vi "Script Editor.vi"(3 "error in (no error)":errorcluster) -> (0 "error out":errorcluster)   [LabVIEW 2011]
uses:
  Strict Type Controls/Settings Operation.ctl
  <userlib>/_OpenG.lib/comparison/comparison.llb/Boolean Changed__ogtk.vi
  Instance           1 21Saved   Script Editor .vi
  Instance           2 21Saved   Script Editor .vi
panel:
  out "Quit":bool
  in  "Update":bool
  in  "Remove":bool
  in  "Add":bool
  in  "Save As":bool
  in  "Save":bool
  in  "Open":bool
  in  "New":bool
  in  "Param 2":dbl
  in  "Param 1":dbl
  in  "Command":string(combo)
  in  "Comment":string
  in  "Script":i32(listbox)
  out "File Name":string
  out "Progress":u8(slide) scale=0.0..100.0
  # "App Designed For:"
  # "Web: www.jambhekar.com\nEmail: tushar@jambhekar.com\nCell: +919970168164"
  # "App Designed By:"
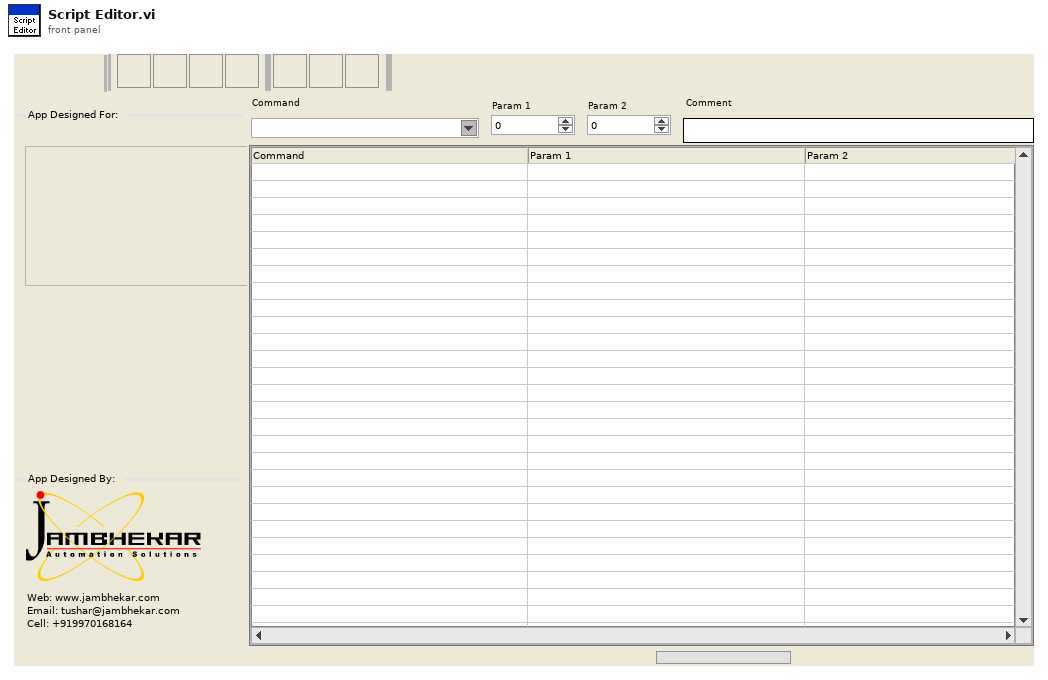
[diagram p1: front panel]
types:
  T1 = enum32{"Invalid", "Standard", "Closed", "Hidden", "Minimized", "Maximized"}
  T2 = typedef "Settings Operation.ctl" = enum8{"Get Value", "Set Value", "Read File", "Write File", "Write Stored Value"}
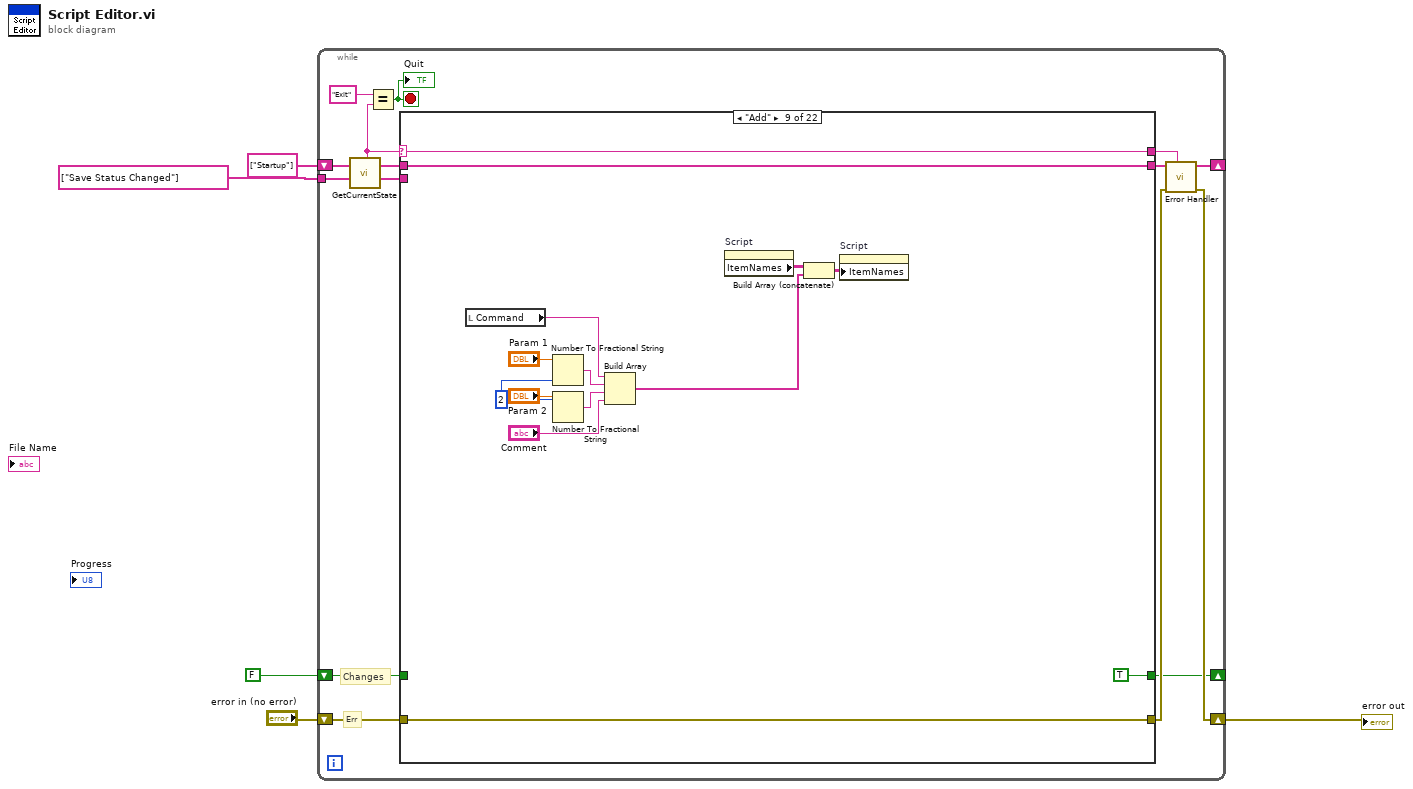
[diagram p0: block diagram]
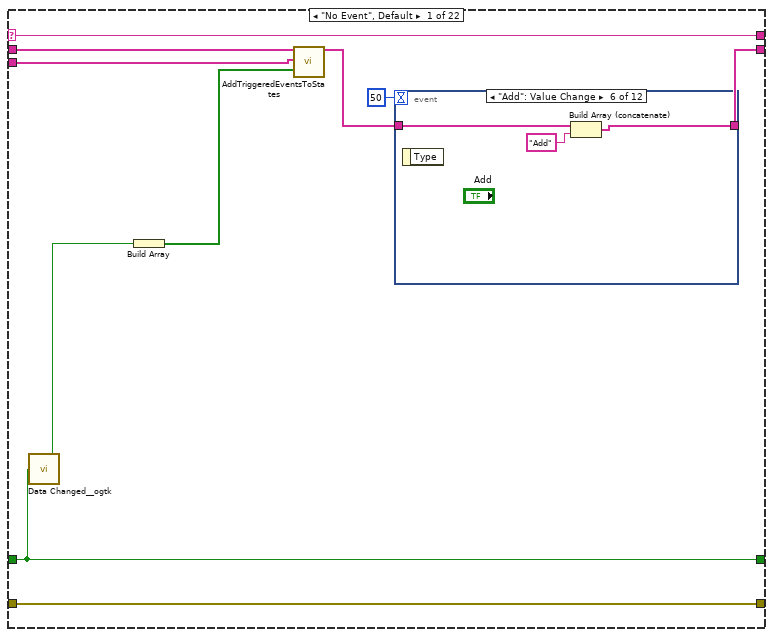
[diagram p2: hidden frame]
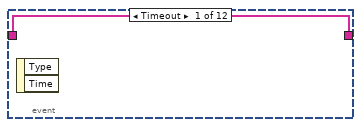
[diagram p3: hidden frame]
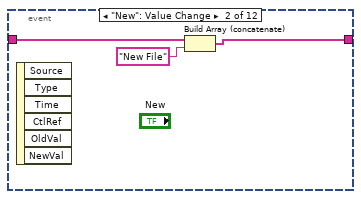
[diagram p4: hidden frame]
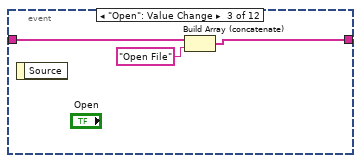
[diagram p5: hidden frame]
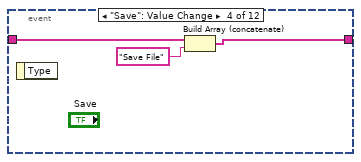
[diagram p6: hidden frame]
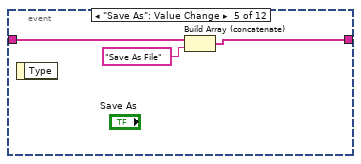
[diagram p7: hidden frame]
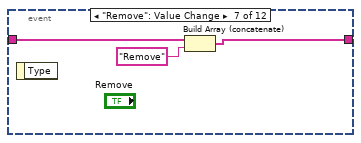
[diagram p8: hidden frame]
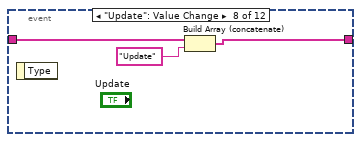
[diagram p9: hidden frame]
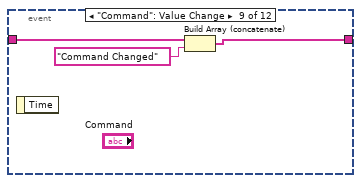
[diagram p10: hidden frame]
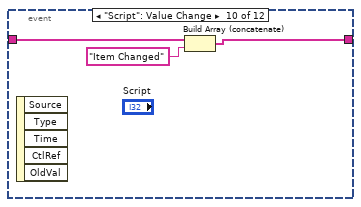
[diagram p11: hidden frame]
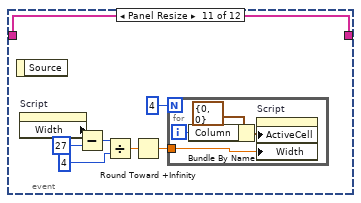
[diagram p12: hidden frame]
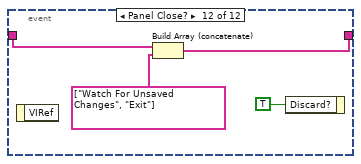
[diagram p13: hidden frame]
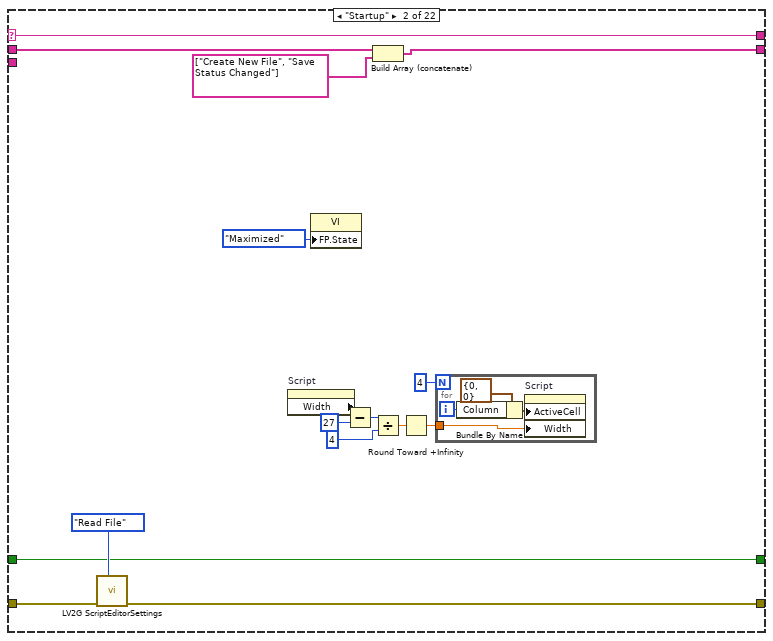
[diagram p14: hidden frame]
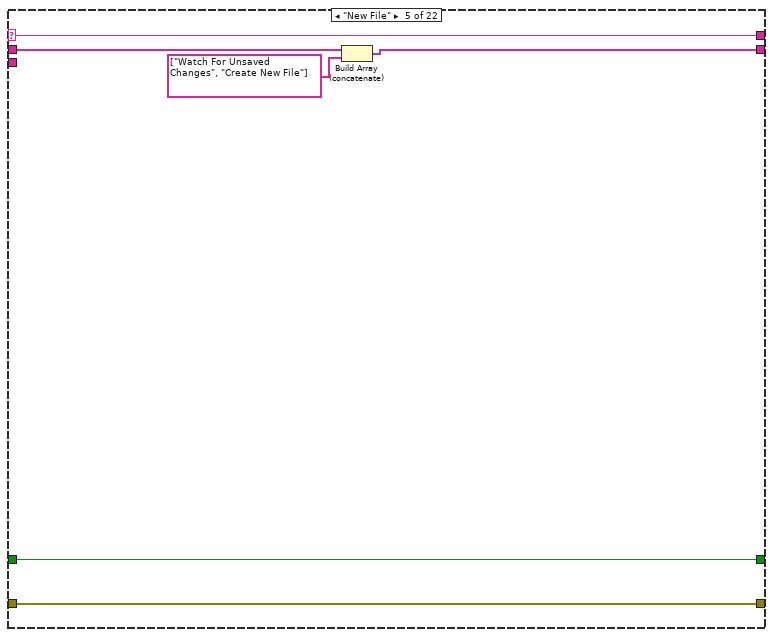
[diagram p17: hidden frame]
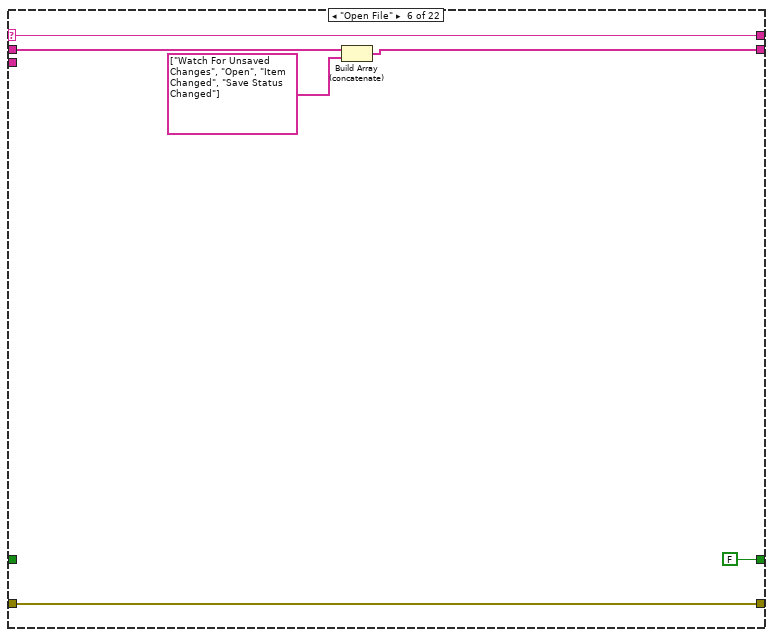
[diagram p18: hidden frame]
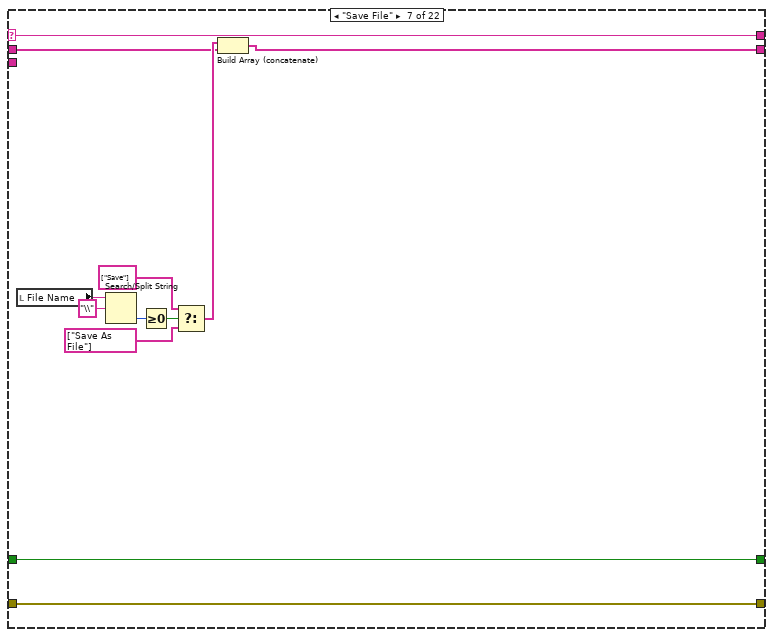
[diagram p19: hidden frame]
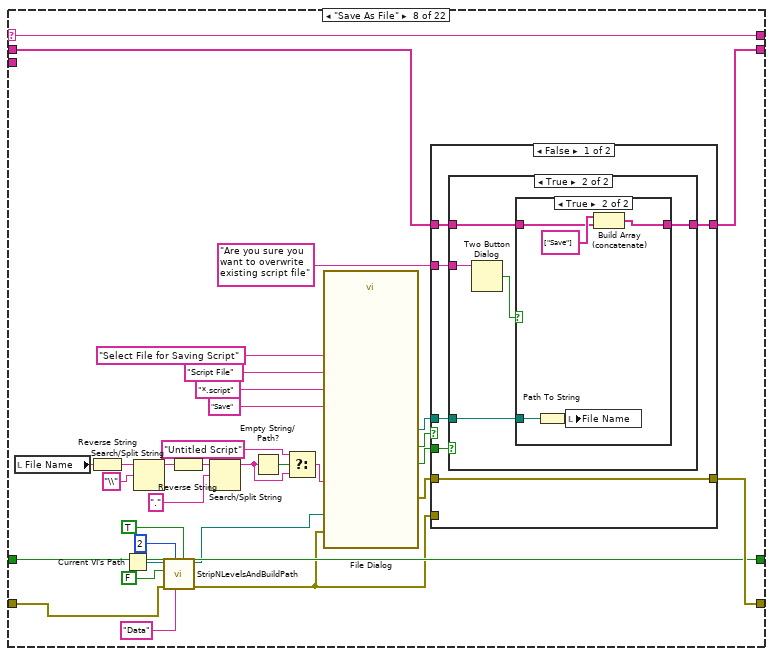
[diagram p20: hidden frame]
diagram:
  n1 = while {
    shift-right: [w13] -> _
    shift-left: string[] ["Startup"] ("State Array Out") -> [w19]
    tunnel: string[] ["Save Status Changed"] ("State Array Out") -> [w17]
    shift-right: [w10] -> w1
    shift-left: "error in (no error)" -> [w14]
    shift-right: [w7] -> _
    shift-left: FALSE -> [w8]
    stop <- w15 stop-if-true
    # "Changes"
    # "Err"
    n2 = call "GetCurrentState.vi"("State Array In"=w19) -> ("Current State"=w6:string, "State Array Out"=w18:string[])  [unwired: 1 in, 16 out]
    n3 = Equal?(x="Exit", y=w6) -> (x = y?=w15:bool)
    "Quit" <- w15
    n4 = case shown="\"Add\"" w6 {
      selector: w6 -> [w27 w89 w95 w99 w106 w112 w124 w157 w193 w206 w221 w226 w237 w243 w247 w253 w274 w279 w298 w317 w332 w336]
      tunnel: w18 -> [w29 w86 w97 w101 w103 w110 w116 w138 w195 w208 w223 w228 w234 w245 w249 w255 w266 w277 w291 w316 w331 w335]
      tunnel: [w22 w85 w97 w101 w102 w109 w115 w137 w195 w208 w223 w228 w233 w245 w249 w255 w265 w276 w290 w316 w331 w335] -> w12
      tunnel: w17 -> [w28 _ _ _ _ _ _ _ _ _ _ _ _ _ _ _ _ _ _ _ _ _]
      tunnel: [w26 w74 w96 w100 w107 w113 w125 w141 w194 w207 w222 w227 w238 w244 w248 w254 w271 w278 w297 w308 w330 errorcluster {"status"=FALSE, "code"=0, "source"=""} ("error in (no error)")] -> w9
      tunnel: w14 -> [w26 w75 w96 w100 w107 w113 w125 w128 w194 w207 w222 w227 w238 w244 w248 w254 w268 w278 w297 w301 w330 _]
      tunnel: [w27 w89 w95 w99 w106 w112 w124 w157 w193 w206 w221 w226 w237 w243 w247 w253 w274 w279 w298 w317 w332 w336] -> w11
      tunnel: w8 -> [w20 w87 w94 w98 w105 _ w114 w134 _ _ _ w225 w236 w242 w246 w251 _ w275 _ _ w329 w334]
      tunnel: [w20 w87 w94 w98 w105 FALSE w114 w134 TRUE TRUE TRUE w225 w236 w242 w246 w251 FALSE w275 FALSE FALSE w329 w334] -> w7
      frame "No Event", Default {
        n5 = call-poly <userlib>:"Data Changed__ogtk.vi"("Boolean"=w20) -> ("Changed"=w21:bool)
        n6 = Build Array(w21) -> (w25:bool[])
        n7 = call "AddTriggeredEventsToStates.vi"("State Array In"=w29, "Event List"=w28, "Event Triggers Array"=w25) -> ("State Array Out"=w23:string[])  [unwired: 16 out]
        n8 = event shown="[5] \"Add\": Value Change" {
          selector: _ -> [_ _ _ _ _ _ _ _ _ _ _ _]
          dyn-events: _ -> [_ _ _ _ _ _ _ _ _ _ _ _]
          timeout: 50 -> [_ _ _ _ _ _ _ _ _ _ _ _]
          tunnel: w23 -> [w30 w32 w35 w38 w41 w44 w47 w50 w53 w56 w59 w72]
          tunnel: [w30 w31 w34 w37 w40 w43 w46 w49 w52 w55 w59 w70] -> w22
          event Timeout {
            n9 = event-data() -> ()  [unwired: 3 out]
          }
          event "New": Value Change {
            n10 = event-data() -> ()  [unwired: 7 out]
            n11 = Build Array (concatenate)(w32, "New File" ("String")) -> (w31:string[])
          }
          event "Open": Value Change {
            n12 = event-data() -> ()  [unwired: 2 out]
            n13 = Build Array (concatenate)(w35, "Open File" ("String")) -> (w34:string[])
          }
          event "Save": Value Change {
            n14 = event-data() -> ()  [unwired: 2 out]
            n15 = Build Array (concatenate)(w38, "Save File" ("String")) -> (w37:string[])
          }
          event "Save As": Value Change {
            n16 = event-data() -> ()  [unwired: 2 out]
            n17 = Build Array (concatenate)(w41, "Save As File" ("String")) -> (w40:string[])
          }
          event "Add": Value Change {
            n18 = event-data() -> ()  [unwired: 2 out]
            n19 = Build Array (concatenate)(w44, "Add" ("String")) -> (w43:string[])
          }
          event "Remove": Value Change {
            n20 = event-data() -> ()  [unwired: 2 out]
            n21 = Build Array (concatenate)(w47, "Remove" ("String")) -> (w46:string[])
          }
          event "Update": Value Change {
            n22 = event-data() -> ()  [unwired: 2 out]
            n23 = Build Array (concatenate)(w50, "Update" ("String")) -> (w49:string[])
          }
          event "Command": Value Change {
            n24 = event-data() -> ()  [unwired: 2 out]
            n25 = Build Array (concatenate)(w53, "Command Changed" ("String")) -> (w52:string[])
          }
          event "Script": Value Change {
            n26 = event-data() -> ()  [unwired: 6 out]
            n27 = Build Array (concatenate)(w56, "Item Changed" ("String")) -> (w55:string[])
          }
          event Panel Resize {
            n28 = event-data() -> ()  [unwired: 2 out]
            n29 = property on="Script" class="MCListbox (strict)"() -> ("Width"=w60:u32)  [unwired: 2 in, 2 out]
            n30 = Subtract(x=w60, y=u32 27) -> (x-y=w62:u32)
            n31 = Divide(x=w62, y=u32 4) -> (x/y=w64:dbl)
            n32 = Round Toward +Infinity(x=w64) -> (ceil(x): smallest int >= x=w65:dbl)
            n33 = for {
              N: 4 -> [_]
              tunnel: w65 -> [w66]
              i -> [w68]
              n34 = Bundle By Name(cluster=cluster{"Row":i32, "Column":i32} {"Row"=0, "Column"=0} ("Active Cell:Active Cell"), "Column"=w68) -> (w67:cluster{"Row":i32, "Column":i32})
              n35 = property on="Script" class="MCListbox (strict)"("ActiveCell"=w67, "Width"=w66) -> ()  [unwired: 2 in, 2 out]
            }
          }
          event Panel Close? {
            n36 = event-data() -> ()  [unwired: 2 out]
            n37 = Build Array (concatenate)(w72, string[] ["Watch For Unsaved Changes", "Exit"] ("State Array Out")) -> (w70:string[])
            n38 = event-data("Discard?"=TRUE) -> ()  [unwired: 1 in, 1 out]
          }
        }
      }
      frame "Startup" {
        n39 = call "LV2G ScriptEditorSettings.vi"("Operation"=Settings_Operation."Read File", "error in (no error)"=w75) -> ("error out"=w74:errorcluster)  [unwired: 1 in, 8 out]
        n40 = property on="Script" class="MCListbox (strict)"() -> ("Width"=w78:u32)  [unwired: 2 in, 2 out]
        n41 = property class="VI"("FP.State"=T1."Maximized" ("Front Panel Window:State")) -> ()  [unwired: 2 in, 2 out]
        n42 = Subtract(x=w78, y=u32 27) -> (x-y=w80:u32)
        n43 = Build Array (concatenate)(w86, string[] ["Create New File", "Save Status Changed"] ("State Array Out")) -> (w85:string[])
        n44 = Divide(x=w80, y=u32 4) -> (x/y=w82:dbl)
        n45 = Round Toward +Infinity(x=w82) -> (ceil(x): smallest int >= x=w83:dbl)
        n46 = for {
          N: 4 -> [_]
          tunnel: w83 -> [w90]
          i -> [w92]
          n47 = Bundle By Name(cluster=cluster{"Row":i32, "Column":i32} {"Row"=0, "Column"=0} ("Active Cell:Active Cell"), "Column"=w92) -> (w91:cluster{"Row":i32, "Column":i32})
          n48 = property on="Script" class="MCListbox (strict)"("ActiveCell"=w91, "Width"=w90) -> ()  [unwired: 2 in, 2 out]
        }
      }
      frame "Exit" {
      }
      frame "---------------Below are UI Events---------------" {
      }
      frame "New File" {
        n49 = Build Array (concatenate)(w103, string[] ["Watch For Unsaved Changes", "Create New File"] ("State Array Out")) -> (w102:string[])
      }
      frame "Open File" {
        n50 = Build Array (concatenate)(w110, string[] ["Watch For Unsaved Changes", "Open", "Item Changed", "Save Status Changed"] ("State Array Out")) -> (w109:string[])
      }
      frame "Save File" {
        n51 = local read "File Name"() -> (w123:string)
        n52 = Search/Split String(string=w123, search string/char (-)="\\") -> (offset of match=w121:i32)  [unwired: 3 out]
        n53 = Greater Or Equal To 0?(x=w121) -> (x >= 0?=w120:bool)
        n54 = Select(t=string[] ["Save"] ("State Array Out"), s=w120, f=string[] ["Save As File"] ("State Array Out")) -> (s? t:f=w117:string[])
        n55 = Build Array (concatenate)(w117, w116) -> (w115:string[])
      }
      frame "Save As File" {
        n56 = local read "File Name"() -> (w154:string)
        n57 = Reverse String(1:w154) -> (0:w153:string)
        n58 = Current VI's Path() -> (path=w130:path)
        n59 = Search/Split String(string=w153, search string/char (-)="\\") -> (substring before match=w151:string)  [unwired: 3 out]
        n60 = call "StripNLevelsAndBuildPath.vi"("Create Folders"=TRUE, "Build Path"="Data" ("button label"), "Strip Levels"=2, "error in(no error)"=w128, "Is File"=FALSE, "Path In"=w130) -> ("error out"=w127:errorcluster, "Path Out"=w126:path)  [unwired: 4 out]
        n61 = Reverse String(1:w151) -> (0:w150:string)
        n62 = Search/Split String(string=w150, search string/char (-)=".") -> (substring before match=w147:string)  [unwired: 3 out]
        n63 = Empty String/Path?(string/path=w147) -> (empty?=w148:bool)
        n64 = Select(t="Untitled Script", s=w148, f=w147) -> (s? t:f=w145:string)
        n65 = call "File Dialog"("start path"=w126, "prompt"="Select File for Saving Script", "button label"="Save", "default name"=w145, "error in"=w127, "pattern (all files)"="*.script", "pattern label"="Script File") -> ("selected path"=w139:path, "exists"=w136:bool, "cancelled"=w142:bool, "error out"=w140:errorcluster)  [unwired: 5 out]
        n66 = case shown="False" w142 {
          tunnel: [w163 w180] -> w141
          tunnel: w140 -> [w163 _]
          tunnel: w139 -> [w160 _]
          tunnel: w138 -> [w162 w181]
          tunnel: [w161 w181] -> w137
          tunnel: w127 -> [_ w180]
          tunnel: w136 -> [w159 _]
          tunnel: "Are you sure you want to overwrite existing script file" ("prompt") -> [w158 _]
          frame False {
            n67 = case shown="True" w159 {
              tunnel: w162 -> [w167 w173]
              tunnel: [w166 w172] -> w161
              tunnel: w160 -> [w165 w171]
              tunnel: w158 -> [_ w170]
              frame False {
                n68 = Path To String(path=w165) -> (string=w164:string)
                n69 = local write "File Name"(w164) -> ()
                n70 = Build Array (concatenate)(string[] ["Save"] ("State Array Out"), w167) -> (w166:string[])
              }
              frame True {
                n71 = Two Button Dialog(message=w170) -> (T button?=w169:bool)  [unwired: 2 out]
                n72 = case shown="True" w169 {
                  tunnel: w173 -> [w174 w178]
                  tunnel: [w174 w177] -> w172
                  tunnel: w171 -> [_ w176]
                  frame False {
                  }
                  frame True {
                    n73 = Path To String(path=w176) -> (string=w175:string)
                    n74 = local write "File Name"(w175) -> ()
                    n75 = Build Array (concatenate)(string[] ["Save"] ("State Array Out"), w178) -> (w177:string[])
                  }
                }
              }
            }
          }
          frame True {
          }
        }
      }
      frame "Add" {
        w182 = i16 2 ("precision (6)")
        n76 = local read "Command"() -> (w187:string)
        n77 = Number To Fractional String(number="Param 1", precision (6)=w182) -> (F-format string=w186:string)  [unwired: 2 out]
        n78 = Number To Fractional String(number="Param 2", precision (6)=w182) -> (F-format string=w185:string)  [unwired: 2 out]
        n79 = Build Array(w187, w186, w185, "Comment") -> (w183:string[])
        n80 = property on="Script" class="MCListbox (strict)"() -> ("ItemNames"=w192:string[][])  [unwired: 2 in, 2 out]
        n81 = Build Array (concatenate)(w192, w183) -> (w191:string[][])
        n82 = property on="Script" class="MCListbox (strict)"("ItemNames"=w191) -> ()  [unwired: 2 in, 2 out]
      }
      frame "Remove" {
        n83 = property on="Script" class="MCListbox (strict)"() -> ("ItemNames"=w205:string[][])  [unwired: 2 in, 2 out]
        n84 = local read "Script"() -> (w204:i32)
        n85 = Delete From Array(array=w205, index (row)=w204) -> (array with subset deleted=w201:string[][])  [unwired: 2 in, 1 out]
        n86 = property on="Script" class="MCListbox (strict)"("ItemNames"=w201) -> ("Value"=w202:i32)  [unwired: 2 in, 2 out]
        n87 = Array Size(array=w201) -> (size(s)=w200:i32[])
        n88 = Index Array(array=w200) -> (element=w199:i32)  [unwired: 1 in]
        n89 = Greater Or Equal To 0?(x=w202) -> (x >= 0?=w203:bool)
        n90 = Decrement(x=w199) -> (x-1=w198:i32)
        n91 = Select(t=w202, s=w203, f=w198) -> (s? t:f=w197:i32)
        n92 = local write "Script"(w197) -> ()
      }
      frame "Update" {
        w209 = i16 2 ("precision (6)")
        n93 = local read "Command"() -> (w216:string)
        n94 = local read "Comment"() -> (w211:string)
        n95 = local read "Param 1"() -> (w213:dbl)
        n96 = local read "Param 2"() -> (w212:dbl)
        n97 = Number To Fractional String(number=w213, precision (6)=w209) -> (F-format string=w215:string)  [unwired: 2 out]
        n98 = Number To Fractional String(number=w212, precision (6)=w209) -> (F-format string=w214:string)  [unwired: 2 out]
        n99 = Build Array(w216, w215, w214, w211) -> (w210:string[])
        n100 = property on="Script" class="MCListbox (strict)"() -> ("ItemNames"=w220:string[][])  [unwired: 2 in, 2 out]
        n101 = local read "Script"() -> (w218:i32)
        n102 = Replace Array Subset(array=w220, new element=w210, index (row)=w218) -> (w219:string[][])  [unwired: 1 in]
        n103 = property on="Script" class="MCListbox (strict)"("ItemNames"=w219) -> ()  [unwired: 2 in, 2 out]
      }
      frame "Command Changed" {
        n104 = local read "Command"() -> (w224:string)
        n105 = case shown="\"Set Relays\", \"Wait\"" w224 {
          frame Default {
            n106 = property on="Param 2" class="DigNum (strict)"("Visible"=TRUE, "Value"=0.0 ("Param 2")) -> ()  [unwired: 2 in, 2 out]
          }
          frame "Read DMM" {
            n107 = property on="Param 2" class="DigNum (strict)"("Visible"=TRUE) -> ()  [unwired: 2 in, 2 out]
          }
          frame "Set Relays", "Wait" {
            n108 = property on="Param 2" class="DigNum (strict)"("Visible"=FALSE) -> ()  [unwired: 2 in, 2 out]
          }
        }
      }
      frame "Open Windows Script" {
        n109 = Build Array (concatenate)(w234, string[] ["Watch For Unsaved Changes", "Open Queued File", "Item Changed"] ("State Array Out")) -> (w233:string[])
      }
      frame "Save Status Changed" {
        n110 = Select(t="Script Editor *", s=w242, f="Script Editor") -> (s? t:f=w239:string)
        n111 = property class="VI"("Front Panel.Title"=w239) -> ()  [unwired: 2 in, 2 out]
      }
      frame "---------------Below are Subroutine states---------------" {
      }
      frame "Item Changed" {
        n112 = property on="Script" class="MCListbox (strict)"() -> ("ItemNames"=w252:string[][])  [unwired: 2 in, 2 out]
        n113 = local read "Script"() -> (w250:i32)
        n114 = case shown="0.." w250 {
          selector: w250 -> [_ w256]
          tunnel: w252 -> [_ w264]
          frame ..-1 {
          }
          frame 0.. {
            n115 = Index Array(array=w264, index (row)=w256) -> (element=w263:string[])  [unwired: 1 in]
            n116 = Index Array(array=w263) -> (element #1=w262:string, element #2=w260:string, element #3=w259:string, element #4=w261:string)  [unwired: 4 in]
            n117 = Fract/Exp String To Number(string=w260) -> (number=w258:dbl)  [unwired: 4 out]
            n118 = Fract/Exp String To Number(string=w259) -> (number=w257:dbl)  [unwired: 4 out]
            n119 = local write "Command"(w262) -> ()
            n120 = local write "Param 1"(w258) -> ()
            n121 = local write "Param 2"(w257) -> ()
            n122 = local write "Comment"(w261) -> ()
          }
        }
      }
      frame "Save" {
        n123 = local read "File Name"() -> (w273:string)
        n124 = property on="Script" class="MCListbox (strict)"() -> ("ItemNames"=w269:string[][])  [unwired: 2 in, 2 out]
        n125 = String To Path(string=w273) -> (path=w270:path)
        n126 = call "WriteScriptFile.vi"("error in (no error)"=w268, "Script"=w269, "Path"=w270) -> ("error out"=w271:errorcluster)  [unwired: 7 in, 1 out]
        n127 = Build Array (concatenate)(w266, "Save Status Changed" ("String")) -> (w265:string[])
      }
      frame "Watch For Unsaved Changes" {
        n128 = case shown="True" w275 {
          tunnel: [w280 w281] -> w276
          tunnel: w277 -> [w280 w282]
          frame False {
          }
          frame True {
            n129 = Build Array (concatenate)("Save File", w282) -> (w283:string[])
            n130 = Two Button Dialog(message="Do you want to save Changes before proceeding?" ("String"), 1:"No", 2:"Yes") -> (T button?=w285:bool)
            n131 = Select(t=w283, s=w285, f=w282) -> (s? t:f=w281:string[])
          }
        }
      }
      frame "Create New File" {
        n132 = local write "Command"("Read DMM" ("String")) -> ()
        n133 = local write "File Name"("Untitled Script" ("t")) -> ()
        n134 = property on="Script" class="MCListbox (strict)"("ItemNames"=string[][] [] ("Item Names"), "Value"=-1 ("Script")) -> ()  [unwired: 2 in, 2 out]
        n135 = Build Array (concatenate)(string[] ["Command Changed", "Item Changed"] ("State Array Out"), w291) -> (w290:string[])
      }
      frame "Open" {
        n136 = Current VI's Path() -> (path=w303:path)
        n137 = call "StripNLevelsAndBuildPath.vi"("Create Folders"=TRUE, "Build Path"="Data" ("button label"), "Strip Levels"=2, "error in(no error)"=w301, "Is File"=FALSE, "Path In"=w303) -> ("error out"=w300:errorcluster, "Path Out"=w299:path)  [unwired: 4 out]
        n138 = call "File Dialog2"("start path"=w299, "prompt"="Select Script to Open", "button label"="Open", "error in"=w300, "pattern (all files)"="*.script", "pattern label"="Script File") -> ("selected path"=w307:path, "cancelled"=w310:bool, "error out"=w309:errorcluster)  [unwired: 1 in, 6 out]
        n139 = case shown="False" w310 {
          tunnel: [w327 w328] -> w308
          tunnel: w309 -> [w325 _]
          tunnel: w300 -> [_ w328]
          tunnel: w307 -> [w324 _]
          frame False {
            n140 = call "ReadScriptFile.vi"("error in (no error)"=w325, "File"=w324) -> ("error out"=w327:errorcluster, "Script"=w323:string[][], "#Rows"=w322:i32)  [unwired: 1 in, 6 out]
            n141 = Path To String(path=w324) -> (string=w326:string)
            n142 = Greater Than 0?(x=w322) -> (x > 0?=w321:bool)
            n143 = Select(t=0 ("Script"), s=w321, f=-1 ("Script")) -> (s? t:f=w320:i32)
            n144 = local write "File Name"(w326) -> ()
            n145 = property on="Script" class="MCListbox (strict)"("Value"=w320, "ItemNames"=w323) -> ()  [unwired: 2 in, 2 out]
          }
          frame True {
          }
        }
      }
      frame "---------------Below are Error Handling VIs---------------" {
        # "This State will never Execute\nIt is added just for improving code readability please do not remove this case"
      }
      frame "Error" {
      }
    }
    n146 = call "Error Handler.vi"("Current State"=w11, "error in (no error)"=w9, "Msg Queue In"=w12) -> ("error out"=w10:errorcluster, "Msg Queue Out"=w13:string[])  [unwired: 7 out]
  }
  "error out" <- w1
